vi "Auto-Indexing Tunels.vi"() -> ()   [LabVIEW 2020]
panel:
  out "Input Tunnel Result (Auto Index)":dbl
  out "Current Iteration":i32
  out "Output Tunnel Result":i32[](array[numeric])
  in  "1D DBL Array Input":dbl[](array[numeric])=[25.0, 50.0, 75.0, 100.0, 125.0, 150.0, 175.0, 200.0, 225.0, 250.0, 275.0, 300.0]
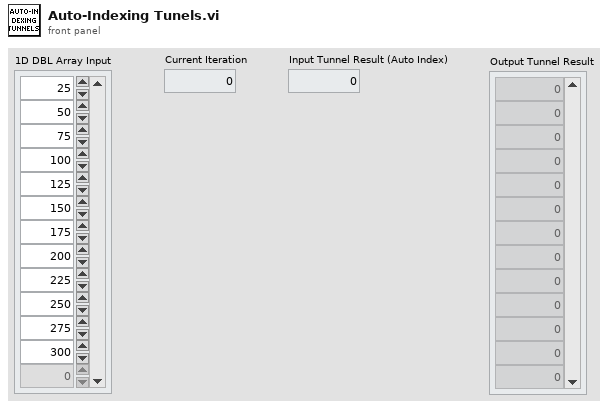
[diagram p1: front panel]
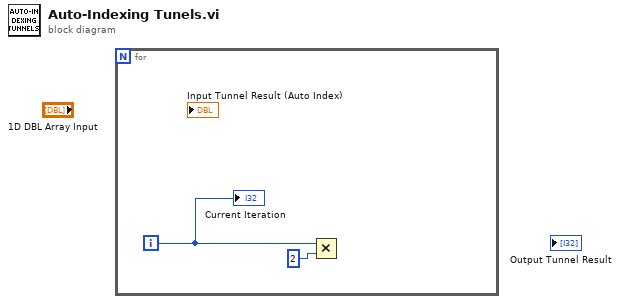
[diagram p0: block diagram]
diagram:
  n1 = for {
    i -> [w2]
    n2 = Multiply(x=w2, y=2) -> ()  [unwired: 1 out]
    "Current Iteration" <- w2
  }
